vi "Sub_Followline.vi"() -> (0 "0 or 8?":bool, 1 "Abweichung\nMittellinie":dbl=1.0, 3 "Linefollow_Array":bool[](array[boolean]))   [LabVIEW 2016]
uses:
  <vilib>/myRIO/Instrument Drivers/Onboard IO/DIO/typedefs/DIO Reference.ctl
  <vilib>/myRIO/Common/Instrument Driver Framework/Utilities/typedefs/myRIO Generic Hardware Reference.ctl
  <vilib>/myRIO/Common/Instrument Driver Framework/Utilities/typedefs/Hardware Version Enum.ctl
  <vilib>/myRIO/Common/Instrument Driver Framework/Utilities/typedefs/myRIO v1.0 Reference.ctl
  <vilib>/myRIO/Common/Instrument Driver Framework/Utilities/typedefs/Generic FPGA Reference.ctl
  <vilib>/myRIO/Common/Instrument Driver Framework/myRIO v1.0/DIO/typedefs/DIO Channels List.ctl
  <vilib>/myRIO/Common/Instrument Driver Framework/myRIO v1.0/DIO/typedefs/DIO Channels Enum.ctl
  <vilib>/userdefined/High Color/nirio_resource_hc.ctl
  <vilib>/myRIO/Common/Instrument Driver Framework/Utilities/vis/Is FPGA Ref Available.vi
  <vilib>/myRIO/Common/Instrument Driver Framework/myRIO v1.0/DIO/vis/myRIO v1.1 Open DIO.vi
  <vilib>/myRIO/Instrument Drivers/Onboard IO/DIO/vis/Read.vi
  <vilib>/myRIO/Common/Instrument Driver Framework/Utilities/vis/Validate Channels.vi
  <vilib>/myRIO/Common/Instrument Driver Framework/myRIO v1.0/DIO/vis/myRIO v1.0 Reserve DIO.vi
  <vilib>/myRIO/Common/Instrument Driver Framework/myRIO v1.0/Resource Manager/vis/myRIO v1.0 Reserve Channel List.vi
  <vilib>/myRIO/Common/Instrument Driver Framework/myRIO v1.0/DIO/vis/myRIO v1.0 Build MUX Configuration DIO.vi
  <vilib>/myRIO/Common/Instrument Driver Framework/myRIO v1.0/Resource Manager/vis/myRIO v1.0 Reserve Channel.vi
  <vilib>/myRIO/Common/Instrument Driver Framework/myRIO v1.0/Resource Manager/vis/myRIO v1.0 Unreserve Channel.vi
  <vilib>/myRIO/Common/Instrument Driver Framework/myRIO v1.0/Resource Manager/vis/myRIO v1.0 Create Configuration List.vi
  <vilib>/myRIO/Common/Instrument Driver Framework/myRIO v1.0/Resource Manager/vis/myRIO v1.0 Build Mutex Name.vi
  <vilib>/Utility/VariantDataType/GetNumericInfo.vi
  <vilib>/Utility/error.llb/Error Cluster From Error Code.vi
  <vilib>/myRIO/Common/Instrument Driver Framework/myRIO v1.0/myRIO v1.1 Open.vi
  <vilib>/myRIO/Common/Instrument Driver Framework/Utilities/vis/IO Manager.vi
  <vilib>/myRIO/Common/Instrument Driver Framework/Utilities/vis/Configuration Manager.vi
  <vilib>/myRIO/Common/Instrument Driver Framework/myRIO v1.0/Resource Manager/vis/myRIO v1.0 Configure IO.vi
  <vilib>/myRIO/Common/Instrument Driver Framework/myRIO v1.0/myRIO v1.0 Close.vi
  <vilib>/myRIO/Common/Instrument Driver Framework/myRIO v1.0/DIO/vis/myRIO v1.0 Read DIO.vi
  <vilib>/myRIO/Express VI/Onboard IO/DI/DI Express VI.xnode
  <vilib>/myRIO/Instrument Drivers/Onboard IO/DIO/vis/myRIO DIO Open.xnode
  <vilib>/myRIO/Instrument Drivers/Onboard IO/DIO/DIO.lvlib
panel:
  in  "Sensorarray\nZusatzwerte":dbl[](array[numeric])=[4.0, 3.0, 2.0, 1.0, -1.0, -2.0, -3.0, -4.0]
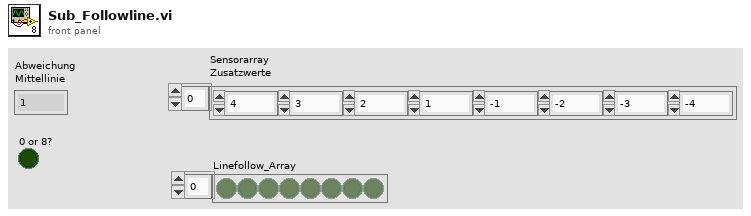
[diagram p1: front panel]
types:
  T1 = cluster{"A/DIO0 (Pin 11)":bool, "A/DIO1 (Pin 13)":bool, "A/DIO2 (Pin 15)":bool, "A/DIO3 (Pin 17)":bool, "A/DIO4 (Pin 19)":bool, "A/DIO5 (Pin 21)":bool, "A/DIO6 (Pin 23)":bool, "A/DIO7 (Pin 25)":bool}
  T2 = cluster{"A/DIO0 (Pin 11)":i16, "A/DIO1 (Pin 13)":i16, "A/DIO2 (Pin 15)":i16, "A/DIO3 (Pin 17)":i16, "A/DIO4 (Pin 19)":i16, "A/DIO5 (Pin 21)":i16, "A/DIO6 (Pin 23)":i16, "A/DIO7 (Pin 25)":i16}
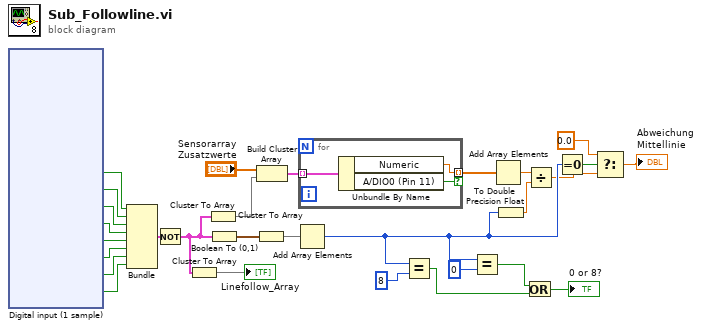
[diagram p0: block diagram]
diagram:
  n1 = xnode "Digital input (1 sample)"() -> ("A/DIO0 (Pin 11)"=w11:bool, "A/DIO1 (Pin 13)"=w12:bool, "A/DIO2 (Pin 15)"=w13:bool, "A/DIO3 (Pin 17)"=w14:bool, "A/DIO4 (Pin 19)"=w15:bool, "A/DIO5 (Pin 21)"=w16:bool, "A/DIO6 (Pin 23)"=w17:bool, "A/DIO7 (Pin 25)"=w18:bool)  [unwired: 1 in, 1 out]
  n2 = Bundle("A/DIO0 (Pin 11)"=w11, "A/DIO1 (Pin 13)"=w12, "A/DIO2 (Pin 15)"=w13, "A/DIO3 (Pin 17)"=w14, "A/DIO4 (Pin 19)"=w15, "A/DIO5 (Pin 21)"=w16, "A/DIO6 (Pin 23)"=w17, "A/DIO7 (Pin 25)"=w18) -> (w6:T1)  [unwired: 1 in]
  n3 = Not(x=w6) -> (.not. x?=w28:T1)
  n4 = Cluster To Array(cluster=w28) -> (array=→"Linefollow_Array":bool[])
  n5 = Cluster To Array(cluster=w28) -> (array=w7:bool[])
  n6 = Boolean To (0,1)(Boolean=w28) -> (0, 1=w20:T2)
  n7 = Cluster To Array(cluster=w20) -> (array=w21:i16[])
  n8 = Build Cluster Array("Sensorarray\nZusatzwerte", w7) -> (w8:cluster{"Numeric":dbl, "A/DIO0 (Pin 11)":bool}[])
  n9 = Add Array Elements(numeric array=w21) -> (sum=w23:i16)
  n10 = for {
    tunnel: w8 -> [w32] mode=indexing
    tunnel: [w31] -> w10 mode=indexing if=w30
    n11 = Unbundle By Name(w32) -> ("Numeric"=w31:dbl, "A/DIO0 (Pin 11)"=w30:bool)
  }
  n12 = Equal?(x=w23, y=i16 8) -> (x = y?=w25:bool)
  n13 = Equal?(x=w23, y=i16 0) -> (x = y?=w26:bool)
  n14 = Add Array Elements(numeric array=w10) -> (sum=w19:dbl)
  n15 = To Double Precision Float(number=w23) -> (double precision float=w29:dbl)
  n16 = Or(x=w26, y=w25) -> (x .or. y?=→"0 or 8?":bool)
  n17 = Divide(x=w19, y=w29) -> (x/y=w3:dbl)
  n18 = Equal To 0?(x=w23) -> (x = 0?=w1:bool)
  n19 = Select(t=0.0, s=w1, f=w3) -> (s? t:f=→"Abweichung\nMittellinie":dbl)
